vi "students-estimator.vi"() -> (0 "Estimator Script Error":errorcluster, 1 "Estimator State Space Object":T2 {"Transport Delay" format="%.2f"; "D" format="%#.2g"; "C" format="%#.2g"; "B" format="%#.2g"; "A" format="%#.2g"; "properties"."Sampling Time" format="%#.6p"; "properties"."Output Delays" format="%.4f"; "properties"."Input Delays" format="%.4f"}, 2 "State Feedback Gain (K)":T1, 3 "Input Scaling (Nbar)":dbl)   [LabVIEW 2013]
uses:
  <vilib>/addons/Control Design/_Model Construction/Model Typedefs.llb/CD State Space Model (MIMO).ctl
  <vilib>/addons/Control Design/_Model Construction/Model Typedefs.llb/CD General Elements.ctl
  <vilib>/Analysis/Matrix/Datatypes/RealMatrix.ctl
  <vilib>/imath/engines/lvmath2/RunTimeEngine/ErrorHandling/NIMS_Finalize Error.vi
  <vilib>/Analysis/Matrix/Numeric/Conversions/Array To Matrix - RA2.vi
  <vilib>/imath/engines/lvmath2/RunTimeEngine/NodeEndStatement/NIMS_NodeEndStatement_Get Vector.vi
  <instcachedir>/0/NIMS_NodeEndStatement_Get Vector_BE4364D373AE46158CA0B14DEB6F98C8.lvgen/NIMS_NodeEndStatement_Get Vector_BE4364D373AE46158CA0B14DEB6F98C8_001.vi
  <vilib>/imath/engines/lvmath/Functions/Error Handling/MergeErrorsWrapper.vi
  <vilib>/imath/engines/lvmath2/RunTimeEngine/NodeEndStatement/NIMS_NodeEndStatement_Output.vi
  <instcachedir>/0/NIMS_NodeEndStatement_Output_53EC0D466D134D7ABD903AC30B43404B.lvgen/NIMS_NodeEndStatement_Output_53EC0D466D134D7ABD903AC30B43404B_000.vi
  <instcachedir>/0/NIMS_NodeEndStatement_Output_53EC0D466D134D7ABD903AC30B43404B.lvgen/NIMS_NodeEndStatement_Output_53EC0D466D134D7ABD903AC30B43404B_005.vi
  <instcachedir>/0/NIMS_NodeEndStatement_Output_53EC0D466D134D7ABD903AC30B43404B.lvgen/NIMS_NodeEndStatement_Output_53EC0D466D134D7ABD903AC30B43404B_001.vi
  <instcachedir>/0/NIMS_NodeEndStatement_Output_53EC0D466D134D7ABD903AC30B43404B.lvgen/NIMS_NodeEndStatement_Output_53EC0D466D134D7ABD903AC30B43404B_012.vi
  <instcachedir>/0/NIMS_NodeEndStatement_Output_53EC0D466D134D7ABD903AC30B43404B.lvgen/NIMS_NodeEndStatement_Output_53EC0D466D134D7ABD903AC30B43404B_011.vi
  <vilib>/imath/engines/lvmath/Plug In/Control Design/BuiltInFunctions/ss/NIMS_CD_ss(A,B,C,D).vi
  <vilib>/imath/engines/lvmath/Plug In/Control Design/BuiltInFunctions/pzgraph/NIMS_CD_[Poles,Zeros]=pzgraph(SS).vi
  <vilib>/imath/engines/lvmath/Plug In/Control Design/BuiltInFunctions/lqr/NIMS_CD_lqr(A,B,Q,R,N).vi
  <vilib>/imath/engines/lvmath2/RunTimeEngine/BuiltInFunctions/imag/NIMS_imag(Complex).vi
  <instcachedir>/0/NIMS_imag(Complex)_3180D40D00C843A49C2B33397F857BF3.lvgen/NIMS_imag(Complex)_3180D40D00C843A49C2B33397F857BF3_002.vi
  <vilib>/imath/engines/lvmath2/RunTimeEngine/ArithmeticOperatorToken/NIMS_ArithmeticOperator_plus.vi
  <instcachedir>/0/NIMS_ArithmeticOperator_plus_8A46DAFC24D445C9B2C97B626139369E.lvgen/NIMS_ArithmeticOperator_plus_8A46DAFC24D445C9B2C97B626139369E_005.vi
  <vilib>/imathl/engines/lvmath/Functions/Error Handling/Create Error.vi
  <vilib>/imath/engines/lvmath/Plug In/Control Design/BuiltInFunctions/poleplace/NIMS_CD_poleplace(A,B,poles,STR).vi
  <vilib>/imath/engines/lvmath2/RunTimeEngine/RowToken/NIMS_RowToken_M_CV.vi
  <instcachedir>/0/NIMS_RowToken_M_CV_4FFFB80A1A2C4A06BEF1E2564C6BAFA4.lvgen/NIMS_RowToken_M_CV_4FFFB80A1A2C4A06BEF1E2564C6BAFA4_000.vi
  <vilib>/imath/engines/lvmath2/RunTimeEngine/BuiltInFunctions/size/NIMS_I32=size(GM,I32).vi
  <instcachedir>/0/NIMS_I32=size(GM,I32)_0501686D1A7F4581B546512A0CE6115B.lvgen/NIMS_I32=size(GM,I32)_0501686D1A7F4581B546512A0CE6115B_004.vi
  <vilib>/imath/engines/lvmath2/RunTimeEngine/BuiltInFunctions/zeros/NIMS_V=zeros(I32,I32).vi
  <vilib>/imath/engines/lvmath2/RunTimeEngine/BuiltInFunctions/inv/NIMS_inv(GM).vi
  <instcachedir>/0/NIMS_inv(GM)_A6DF8FE880224208AACFE4CF9F659502.lvgen/NIMS_inv(GM)_A6DF8FE880224208AACFE4CF9F659502_000.vi
  <vilib>/imath/engines/lvmath2/RunTimeEngine/ArithmeticOperatorToken/NIMS_ArithmeticOperator_multmx(M,CV).vi
  <instcachedir>/0/NIMS_ArithmeticOperator_multmx(M,CV)_90351521EAFF49D48526FCD9D8E924F7.lvgen/NIMS_ArithmeticOperator_multmx(M,CV)_90351521EAFF49D48526FCD9D8E924F7_002.vi
  <vilib>/imath/engines/lvmath2/RunTimeEngine/ErrorHandling/NIMS_Create Error From Enums.vi
  <vilib>/imath/engines/lvmath2/RunTimeEngine/IndexRead/NIMS M(R2).vi
  <instcachedir>/0/NIMS M(R2)_287818D58BD74005B29FE73CE7602B1A.lvgen/NIMS M(R2)_287818D58BD74005B29FE73CE7602B1A_000.vi
  <vilib>/imath/engines/lvmath2/RunTimeEngine/IndexRead/NIMS M(S).vi
  <instcachedir>/0/NIMS M(S)_B826C018497E4940AE96BD27B540B6FB.lvgen/NIMS M(S)_B826C018497E4940AE96BD27B540B6FB_000.vi
  <vilib>/imath/engines/lvmath2/RunTimeEngine/ArithmeticOperatorToken/NIMS_ArithmeticOperator_multmx(RV,M).vi
  <instcachedir>/0/NIMS_ArithmeticOperator_multmx(RV,M)_814A3E4F784C42EE877A8938CA64A715.lvgen/NIMS_ArithmeticOperator_multmx(RV,M)_814A3E4F784C42EE877A8938CA64A715_001.vi
  <vilib>/Analysis/Matrix/NI_Matrix.lvlib
  <vilib>/addons/Control Design/_Model Construction/NI_LinSys_Model Typedefs.lvlib
panel:
  out "Controller Poles":cdb[](array[numeric])
  out "Observer poles":cdb[](array[numeric])
  out "Open Loop Poles":cdb[](array[numeric])
  out "Open Loop Zeros":cdb[](array[numeric])
  out "K":dbl[](array[numeric])
  out "L":dbl[](array[numeric])
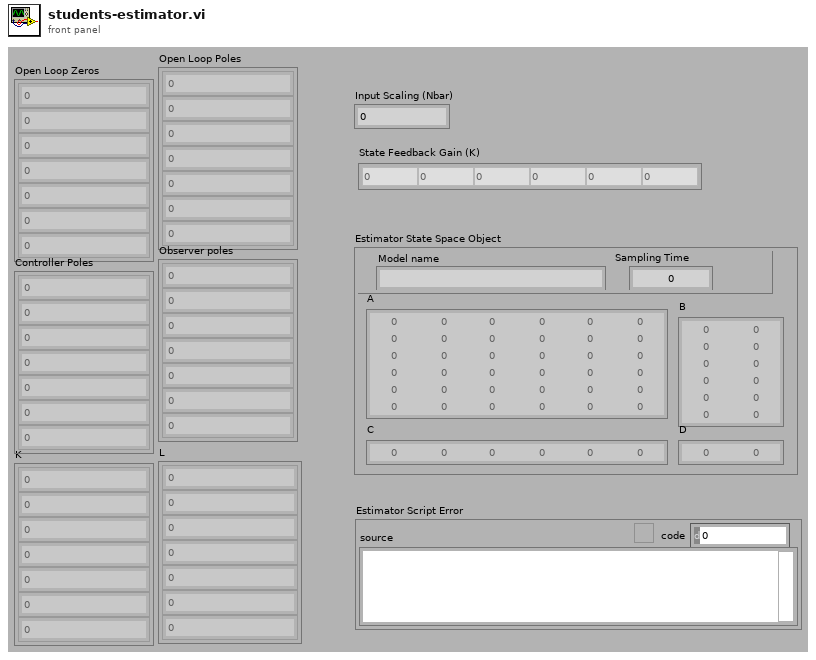
[diagram p1: front panel]
types:
  T1 = typedef "NI_Matrix.lvlib/RealMatrix.ctl" = dbl[][]
  T2 = typedef "NI_LinSys_Model Typedefs.lvlib/CD State Space Model (MIMO).ctl" = cluster{"properties":T3, "A":dbl[][], "B":dbl[][], "C":dbl[][], "D":dbl[][], "StateNames":string[], "Transport Delay":dbl[][]}
  T3 = typedef "NI_LinSys_Model Typedefs.lvlib/CD General Elements.ctl" = cluster{"Model name":string, "Input names":string[], "Output names":string[], "Input Delays":dbl[], "Output Delays":dbl[], "Sampling Time":dbl, "Notes":string}
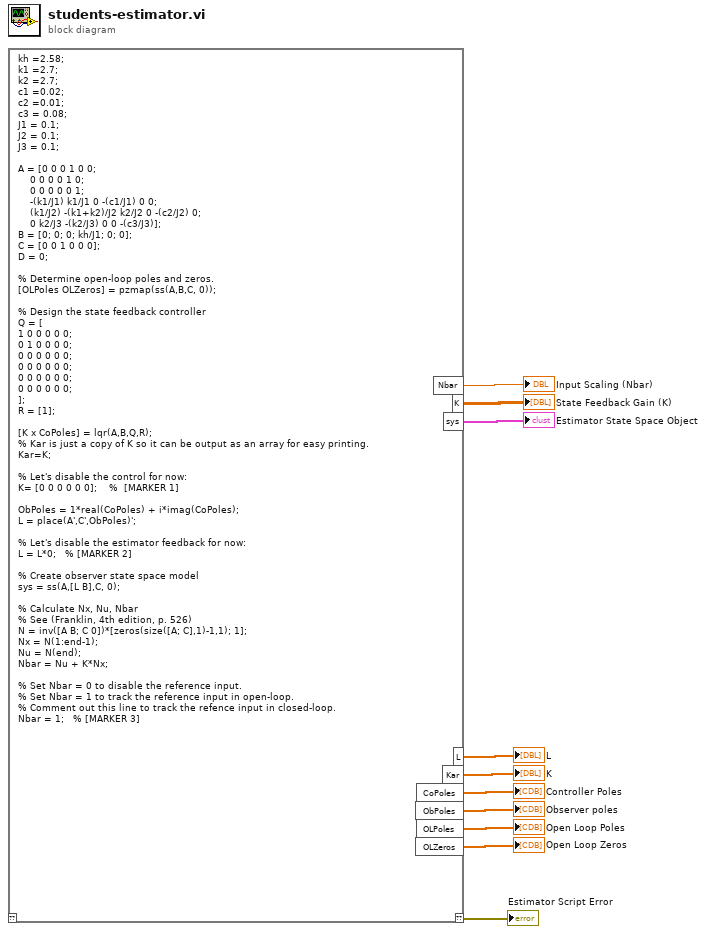
[diagram p0: block diagram]
diagram:
  n1 = mathscript code="kh =2.58;\nk1 =2.7;\nk2 =2.7;\nc1 =0.02;\nc2 =0.01;\nc3 = 0.08;\nJ1 = 0.1;\nJ2 = 0.1;\nJ3 = 0.1;\n\nA = [0 0 0 1 0 0; \n    0 0 0 0 1 0; \n    0 0 0 0 0 1; \n    -(k1/J1) k1/J1 0 -(c1/J1) 0 0;\n    (k1/J2) -(k1+k2)/J2 k2/J2 0 -(c2/J2) 0;\n    0 k2/J3 -(k2/J3) 0 0 -(c3/J3)];\nB = [0; 0; 0; kh/J1; 0; 0];\nC = [0 0 1 0 0 0];\nD = 0;\n\n% Determine open-loop poles and zeros.\n[OLPoles OLZeros] = pzmap(ss(A,B,C, 0));\n\n% Design the state feedback controller\nQ = [\n1 0 0 0 0 0;\n0 1 0 0 0 0;\n0 0 0 0 0 0;\n0 0 0 0 0 0;\n0 0 0 0 0 0;\n0 0 0 0 0 0;\n];\nR = [1];\n\n[K x CoPoles] = lqr(A,B,Q,R);\n% Kar is just a copy of K so it can be output as an array for easy printing.\nKar=K;\n\n% Let's disable the control for now:\nK= [0 0 0 0 0 0];    %  [MARKER 1]\n\nObPoles = 1*real(CoPoles) + i*imag(CoPoles);\nL = place(A',C',ObPoles)';\n\n% Let's disable the estimator feedback for now:\nL = L*0;   % [MARKER 2]\n\n% Create observer state space model\nsys = ss(A,[L B],C, 0);\n\n% Calculate Nx, Nu, Nbar \n% See (Franklin, 4th edition, p. 526)\nN = inv([A B; C 0])*[zeros(size([A; C],1)-1,1); 1];\nNx = N(1:end-1);\nNu = N(end);\nNbar = Nu + K*Nx;\n\n% Set Nbar = 0 to disable the reference input.\n% Set Nbar = 1 to track the reference input in open-loop.\n% Comment out this line to track the refence input in closed-loop.\nNbar = 1;   % [MARKER 3]"() -> ("??"=→"Estimator Script Error":errorcluster, "sys"=→"Estimator State Space Object":T2, "K"=→"State Feedback Gain (K)":T1, "Nbar"=→"Input Scaling (Nbar)":dbl, "L"=→"L":dbl[], "Kar"=→"K":dbl[], "OLPoles"=→"Open Loop Poles":cdb[], "OLZeros"=→"Open Loop Zeros":cdb[], "ObPoles"=→"Observer poles":cdb[], "CoPoles"=→"Controller Poles":cdb[])  [unwired: 1 in]
